vi "xiC - IMAQ - Main.vi"(8 "error in (no error)":errorcluster, 11 "xiCam":refnum<k24>) -> (0 "error out":errorcluster)   [LabVIEW 2013]
doc: "xiControl Main VI. This VI can be used to configure camera parameters and GPI / GPO values.\nThis VI can be called Statically by placing to block diagram or Dynamically with VI server.\n\nCalling this VI with statically connect <b>xiCam</b> parameter for preinited xiCam object, or leave it unwired and the VI automatically initialze a new xiCam object.\n\nDynamic call: Use xiCMNG - Manager VI to handle VI Server call."
uses:
  C:/Projects/Cameras3.x/xiLib/xiLIB_64bit/xiLIB/xiCamLib/API/x64/xiApi.NETX64.dll
  xiLIB_64bit/xiLIB/xiCamLib/API/x64/xiApi.NETX64.dll
  xiCamLib/xiLIB/Typedefs/xiLIB - Control.ctl
  xiCamLib/xiCam/PRM/DOWNSAMPLING_TYPE/DOWNSAMPLING_TYPE.ctl
  xiCamLib/xiCam/PRM/IMG_FORMAT/IMG_DATA_FORMAT.ctl
  xiCamLib/xiCam/PRM/BUFF_POLICY/BUFF_POLICY.ctl
  xiCamLib/xiCam/PRM/TRG_SOURCE/TRG_SOURCE.ctl
  xiCamLib/xiCam/PRM/GPI_MODE/GPI_MODE.ctl
  xiCamLib/xiCam/PRM/GPO_MODE/GPO_MODE.ctl
  xiCamLib/xiCam/PRM/LED_MODE/LED_MODE.ctl
  xiC - IMAQ - States.ctl
  xiC - IMAQ - TreeDisplayType.ctl
  xiCamLib/xiCam/PRM/PRM/PRM_v2.ctl
  xiC - IMAQ - Globals.vi
panel:
  out "Parameter Name":string
  in  "Error":bool=TRUE
  in  "xiControl":T1
  in  "Tree":string(tree)
  out "INFO":string
  in  "RefreshTree":bool
  in  "Stop":bool
  in  "Start":bool
  in  "LOAD":bool
  in  "SAVE":bool
  in  "MANUAL_WB":bool
  in  "SW_TRIG":bool
  in  "GPIO":bool
  out "Image":T9(plugin-control)
  # "xiControl"
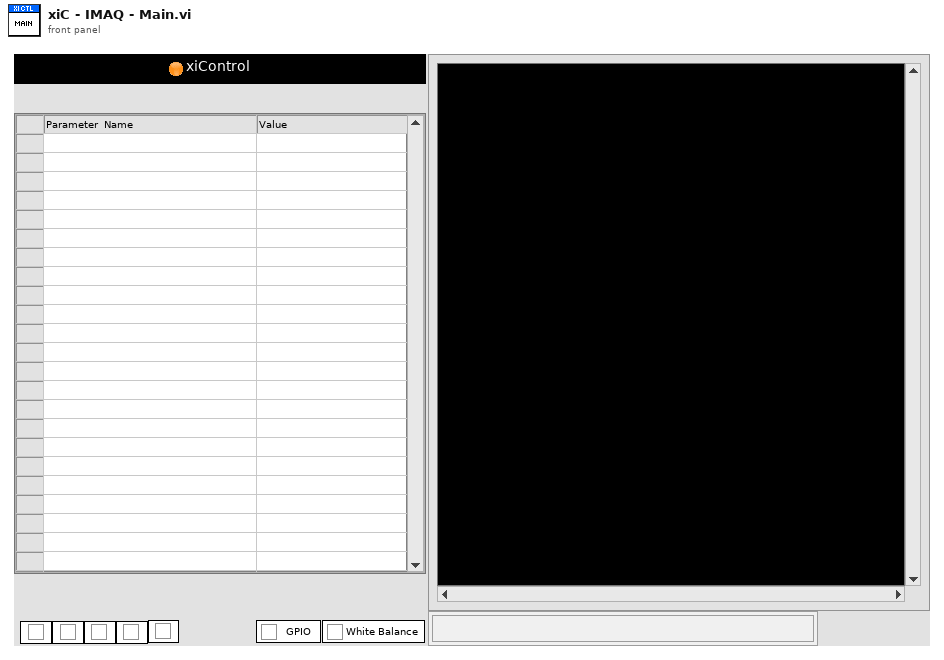
[diagram p1: front panel]
types:
  T1 = typedef "xiLIB - Control.ctl" = cluster{"Int32":i32, "Float":sgl, "String":string, "DOWNSAMPLING_TYPE":T2, "IMG_FORMAT":T3, "BUFF_POLICY":T4, "TRG_SOURCE":T5, "GPI":T6, "GPO":T7, "LED":T8}
  T2 = typedef "DOWNSAMPLING_TYPE.ctl" = enum16{"BINNING", "SKIPPING"}
  T3 = typedef "IMG_DATA_FORMAT.ctl" = enum16{"MONO8", "MONO16", "RGB24", "RGB32", "RGBPLANAR", "RAW8", "RAW16"}
  T4 = typedef "BUFF_POLICY.ctl" = enum16{"UNSAFE", "SAFE"}
  T5 = typedef "TRG_SOURCE.ctl" = enum16{"OFF", "EDGE_RISING", "EDGE_FALLING", "SOFTWARE"}
  T6 = typedef "GPI_MODE.ctl" = enum16{"OFF", "TRIGGER", "EXT_EVENT"}
  T7 = typedef "GPO_MODE.ctl" = enum16{"OFF", "ON", "FRAME_ACTIVE", "FRAME_ACTIVE_NEG", "EXPOSURE_ACTIVE", "EXPOSURE_ACTIVE_NEG"}
  T8 = typedef "LED_MODE.ctl" = enum16{"HEARTBEAT", "TRIGGER_ACTIVE", "EXT_EVENT_ACTIVE", "ACQUSITION", "EXPOSURE_ACTIVE", "FRAME_ACTIVE", "LINK", "OFF", "ON"}
  T9 = typedef "IMAQ Image.ctl" = refnum<image>
  T10 = typedef "xiC - IMAQ - TreeDisplayType.ctl" = enum16{"DEFAULT", "HIDE_MAX_MIN"}
  T11 = typedef "xiC - IMAQ - States.ctl" = enum16{"Idle", "Init", "Exit", "//PRM_UPDATE"}
  T12 = typedef "xiC - IMAQ - Attributes.ctl" = cluster{"Controls":cluster{"VI Ref.":refnum<vi>, "Tree":refnum<vi>, "Info":refnum<vi>, "PRMName":refnum<vi>, "xiControl":refnum<vi>, "Error":refnum<vi>, "SW_TRG":refnum<vi>, "ImageDisplay":refnum<vi>}, "Variables":cluster{"ProcessQ.":refnum<queue>, "Data":bool, "xiCam":refnum<k24>, "Tree_Display_Type":T10}}
  T13 = typedef "PRM_v2.ctl" = enum16{"ACQ_BUFFER_SIZE", "ACQ_FRAME_BURST_COUNT", "ACQ_TIMING_MODE", "ACQ_TRANSPORT_BUFFER_SIZE", "AE_MAX_LIMIT", "AEAG", "AEAG_LEVEL", "API_VERSION", "AG_MAX_LIMIT", "APPLY_CMS", "AUTO_BANDWIDTH_CALCULATION", "AUTO_WB", "AVAILABLE_BANDWIDTH", "AVAILABLE_BANDWIDTH_MAX", "AVAILABLE_BANDWIDTH_MIN", "BPC", "BUFFER_POLICY", "BUFFERS_QUEUE_SIZE", "CC_MATRIX_00", "CC_MATRIX_01", "CC_MATRIX_02", "CC_MATRIX_03", "CC_MATRIX_10", "CC_MATRIX_11", "CC_MATRIX_12", "CC_MATRIX_13", "CC_MATRIX_20", "CC_MATRIX_21", "CC_MATRIX_22", "CC_MATRIX_23", "CC_MATRIX_30", "CC_MATRIX_31", "CC_MATRIX_32", "CC_MATRIX_33", "CHIP_TEMP", "CMS", "COLOR_FILTER_ARRAY", "COOLING", "DEBOUNCE_EN", "DEBOUNCE_POL", "DEBOUNCE_T0", "DEBOUNCE_T1", "DEBUG_LEVEL", "DEFAULT_CC_MATRIX", "DEVICE_INSTANCE_PATH", "DEVICE_MODEL_ID", "DEVICE_NAME", "DEVICE_SN", "DEVICE_TYPE", "DEVICE_USER_ID", "DOWNSAMPLING", "DOWNSAMPLING_MAX", "DOWNSAMPLING_MIN", "DOWNSAMPLING_TYPE", "DRV_VERSION", "EXP_PRIORITY", "EXPOSURE", "EXPOSURE_DIRECT_UPDATE", "EXPOSURE_MAX", "EXPOSURE_MIN", "FFS_FILE_NAME", "FPGA1_VERSION", "FRAMERATE", "FRAMERATE_MAX", "FRAMERATE_MIN", "FREE_FFS_SIZE", "GAIN", "GAIN_DIRECT_UPDATE", "GAIN_MAX", "GAIN_MIN", "GAMMAC", "GAMMAY", "GPI_LEVEL", "GPI_MODE", "GPI_SELECTOR", "GPI_SELECTOR_MAX", "GPI_SELECTOR_MIN", "GPO_MODE", "GPO_SELECTOR", "GPO_SELECTOR_MAX", "GPO_SELECTOR_MIN", "HDR", "HDR_T1", "HDR_T2", "HEIGHT", "HEIGHT_MAX", "HEIGHT_MIN", "HOUSE_TEMP", "IMAGE_DATA_FORMAT", "IMAGE_IS_COLOR", "INPUT_CMS_PROFILE", "IS_COOLED", "IS_DEVICE_EXIST", "KNEEPOINT1", "KNEEPOINT2", "LED_MODE", "LED_SELECTOR", "LED_SELECTOR_MAX", "LED_SELECTOR_MIN", "LIMIT_BANDWIDTH", "LIMIT_BANDWIDTH_MAX", "LIMIT_BANDWIDTH_MIN", "LUT_EN", "LUT_INDEX", "LUT_INDEX_MAX", "LUT_INDEX_MIN", "LUT_VALUE", "LUT_VALUE_MAX", "LUT_VALUE_MIN", "MANUAL_WB", "MCU1_VERSION", "MCU2_VERSION", "OFFSET_X", "OFFSET_X_MAX", "OFFSET_X_MIN", "OFFSET_Y", "OFFSET_Y_MAX", "OFFSET_Y_MIN", "OUTPUT_CMS_PROFILE", "OUTPUT_DATA_BIT_DEPTH", "OUTPUT_DATA_PACKING", "READ_FILE_FFS", "RECENT_FRAME", "SENSOR_DATA_BIT_DEPTH", "SENSOR_MODE", "SENSOR_TAPS", "SHARPNESS", "SHUTTER_TYPE", "TARGET_TEMP", "TRG_DELAY", "TRG_SELECTOR", "TRG_SOFTWARE", "TRG_SOURCE", "USED_FFS_SIZE", "WB_KB", "WB_KG", "WB_KR", "WIDTH", "WIDTH_MAX", "WIDTH_MIN", "WRITE_FILE_FFS", "ACQ_BUFFER_SIZE_UNIT", "ACQ_TRANSPORT_BUFFER_COMMIT", "AEAG_ROI_HEIGHT", "AEAG_ROI_OFFSET_X", "AEAG_ROU_OFFSET_Y", "AEAG_ROI_WIDTH", "API_CONTEXT_LIST", "BINNING_HORIZONTAL", "BINNING_PATTERN", "BINNING_SELECTOR", "BINNING_VERTICAL", "COLUMN_FPN_CORRECTION", "COUNTER_SELECTOR", "COUNTER_VALUE", "DECIMATION_HORIZONTAL", "DECIMATION_PATTERN", "DECIMATION_SELECTOR", "DECIMATION_VERTICAL", "DEVICE_ID", "DEVICE_LOCATION_PATH", "DEVICE_MANIFEST", "DEVICE_RESET", "DEVICE_SENS_SN", "EXPOSURE_BURST_COUNT", "FFS_ACCESS_KEY", "GAIN_SELECTOR", "HW_REVISION", "IMAGE_BLACK_LEVEL", "IMAGE_DATA_BIT_DEPTH", "IMAGE_DATA_FORMAT_RGB32_ALPHA", "IMAGE_PAYLOAD_SIZE", "LENS_APERTURE_VALUE", "LENS_FEATURE", "LENS_FEATURE_SELECTOR", "LENS_FOCAL_LENGTH", "LENS_FOCUS_DISTANCE", "LENS_FOCUS_MOVE", "LENS_FOCUS_MOVEMENT_VALUE", "LENS_MODE", "OUTPUT_DATA_PACKING_TYPE", "SENSOR_CLOCK_FREQ_HZ", "SENSOR_CLOCK_FREQ_INDEX", "SENSOR_FEATURE_SELECTOR", "SENSOR_FEATURE_VALUE", "SENSOR_OUTPUT_CHANNEL_COUNT", "TRANSPORT_PIXEL_FORMAT", "TS_RST_MODE", "TS_RST_SOURCE"}
  T14 = typedef "LVPoint32TypeDef.ctl" = cluster{"Horizontal":i32, "Vertical":i32}
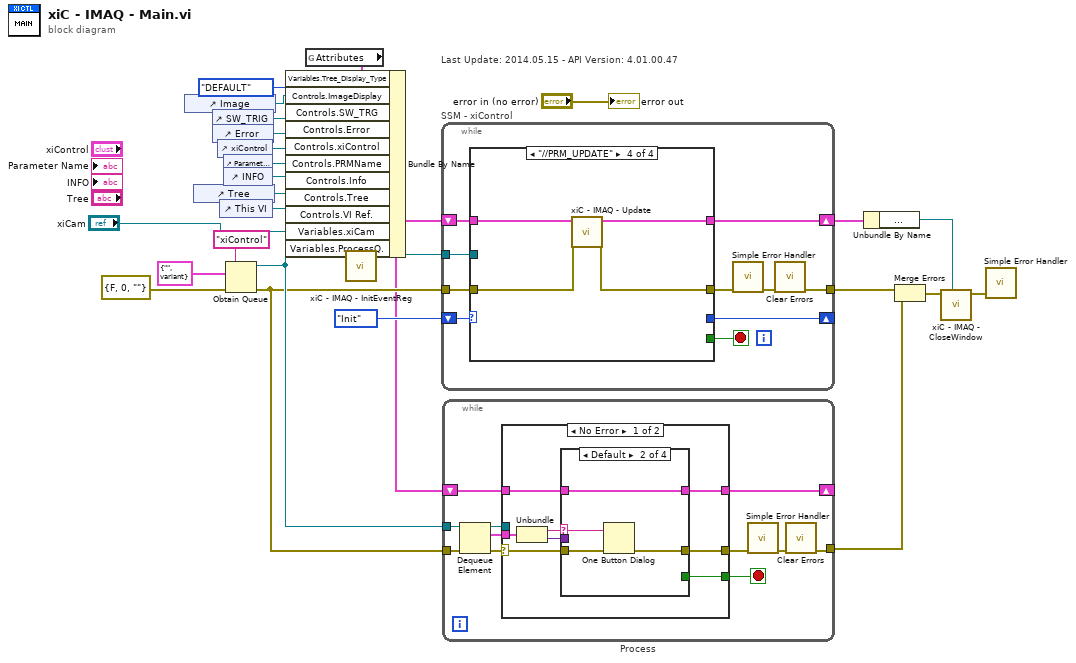
[diagram p0: block diagram]
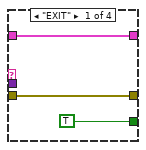
[diagram p2: hidden frame]
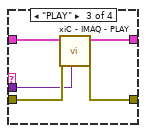
[diagram p3: hidden frame]
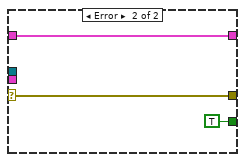
[diagram p5: hidden frame]
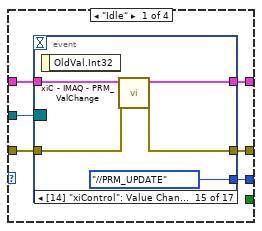
[diagram p6: hidden frame]
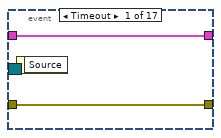
[diagram p7: hidden frame]
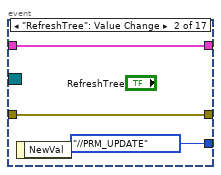
[diagram p8: hidden frame]
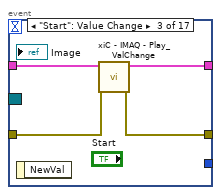
[diagram p9: hidden frame]
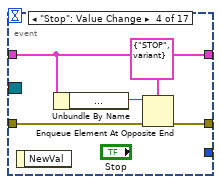
[diagram p10: hidden frame]
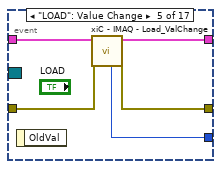
[diagram p11: hidden frame]
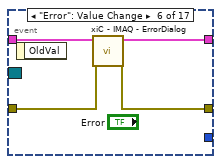
[diagram p12: hidden frame]
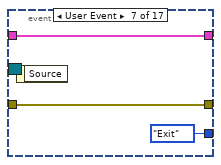
[diagram p13: hidden frame]
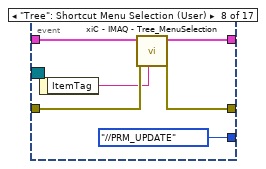
[diagram p14: hidden frame]
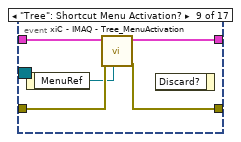
[diagram p15: hidden frame]
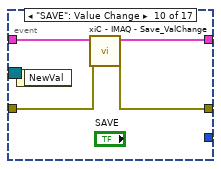
[diagram p16: hidden frame]
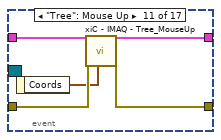
[diagram p17: hidden frame]
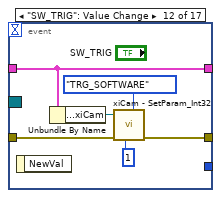
[diagram p18: hidden frame]
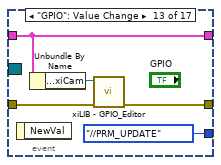
[diagram p19: hidden frame]
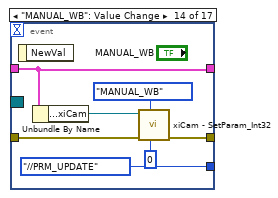
[diagram p20: hidden frame]
diagram:
  # "Last Update: 2014.05.15 - API Version: 4.01.00.47"
  n1 = control-ref of="Image"() -> (w3:refnum<vi>)
  n2 = control-ref of="Tree"() -> (w21:refnum<vi>)
  n3 = control-ref of="SW_TRIG"() -> (w14:refnum<vi>)
  n4 = control-ref of="Error"() -> (w15:refnum<vi>)
  n5 = control-ref of="xiControl"() -> (w1:refnum<vi>)
  n6 = control-ref of="This VI"() -> (w25:refnum<vi>)
  n7 = control-ref of="Parameter Name"() -> (w17:refnum<vi>)
  n8 = control-ref of="INFO"() -> (w18:refnum<vi>)
  n9 = Obtain Queue(name (unnamed)="xiControl", element data type=cluster{"State":string, "Data":variant} {"State"="", "Data"=variant} ("element"), error in (no error)=errorcluster {"status"=FALSE, "code"=0, "source"=""}) -> (queue out=w7:refnum<queue>, error out=w6:errorcluster)  [unwired: 2 in, 1 out]
  n10 = global read "xiC - IMAQ - Globals.vi" "Attributes"() -> (w16:T12)
  n11 = Bundle By Name(cluster=w16, "Variables.Tree_Display_Type"=xiC_-_IMAQ_-_TreeDisplayType."DEFAULT" ("Variables.SAVE_Type"), "Controls.ImageDisplay"=w3, "Controls.SW_TRG"=w14, "Controls.Error"=w15, "Controls.xiControl"=w1, "Controls.PRMName"=w17, "Controls.Info"=w18, "Controls.Tree"=w21, "Controls.VI Ref."=w25, "Variables.xiCam"="xiCam", "Variables.ProcessQ."=w7) -> (w5:T12)
  n12 = call "xiC - IMAQ - InitEventReg.vi"() -> ("EventRegRef"=w13:refnum<event-registration>)  [unwired: 11 in]
  n13 = while "SSM - xiControl" {
    shift-right: [w30] -> _
    shift-left: xiC_-_IMAQ_-_States."Init" ("States") -> [w36]
    shift-right: [w34] -> w23
    shift-left: w5 -> [w35]
    tunnel: w6 -> [w33]
    tunnel: [w31] -> w12
    tunnel: w13 -> [w28]
    stop <- w29 stop-if-true
    n14 = case shown="\"//PRM_UPDATE\"" w36 {
      tunnel: w35 -> [w42 w126 w130 w136]
      tunnel: [w41 w125 w128 w135] -> w34
      tunnel: w33 -> [w40 w124 w129 w134]
      tunnel: [w39 w120 w127 w133] -> w27
      tunnel: [w38 w121 xiC_-_IMAQ_-_States."Exit" ("States") _] -> w30
      tunnel: [_ _ TRUE _] -> w29
      tunnel: w28 -> [w37 _ _ _]
      frame "Idle" {
        n15 = event shown="[14] \"xiControl\": Value Change" {
          selector: w37 -> [_ _ _ _ _ _ _ _ _ _ _ _ _ _ _ _ _]
          dyn-events: _ -> [_ _ _ _ _ _ _ _ _ _ _ _ _ _ _ _ _]
          timeout: _ -> [_ _ _ _ _ _ _ _ _ _ _ _ _ _ _ _ _]
          tunnel: w42 -> [w44 w47 w51 w52 w61 w65 w68 w74 w79 w83 w88 w94 w96 w101 w111 w115 w119]
          tunnel: [w44 w47 w50 w52 w60 w64 w68 w73 w78 w82 w87 w94 w96 w101 w110 w114 w119] -> w41
          tunnel: w40 -> [w43 w46 w49 w54 w59 w63 w67 w72 w77 w81 w86 w92 w99 w103 w109 w113 w117]
          tunnel: [w43 w46 w48 w53 w58 w62 w67 w71 w76 w80 w85 w91 w98 w102 w108 w112 w117] -> w39
          tunnel: [_ xiC_-_IMAQ_-_States."//PRM_UPDATE" ("States") _ _ w57 _ xiC_-_IMAQ_-_States."Exit" ("States") xiC_-_IMAQ_-_States."//PRM_UPDATE" ("States") _ _ _ _ xiC_-_IMAQ_-_States."//PRM_UPDATE" ("States") xiC_-_IMAQ_-_States."//PRM_UPDATE" ("States") xiC_-_IMAQ_-_States."//PRM_UPDATE" ("States") _ xiC_-_IMAQ_-_States."Exit" ("States")] -> w38
          event Timeout {
            n16 = event-data() -> ()  [unwired: 1 in, 1 out]
          }
          event "RefreshTree": Value Change {
            n17 = event-data() -> ()  [unwired: 1 in, 1 out]
          }
          event "Start": Value Change {
            n18 = event-data() -> ()  [unwired: 1 in, 1 out]
            n19 = call "xiC - IMAQ - Play_ValChange.vi"("error in (no error)"=w49, "Attributes In"=w51) -> ("error out"=w48:errorcluster, "Attributes Out"=w50:T12)  [unwired: 8 in]
          }
          event "Stop": Value Change {
            n20 = event-data() -> ()  [unwired: 1 in, 1 out]
            n21 = Unbundle By Name(w52) -> ("Variables.ProcessQ."=w55:refnum<queue>)
            n22 = Enqueue Element At Opposite End(queue=w55, element=cluster{"State":string, "Data":variant} {"State"="STOP", "Data"=variant}, error in (no error)=w54) -> (error out=w53:errorcluster)  [unwired: 1 in, 2 out]
          }
          event "LOAD": Value Change {
            n23 = event-data() -> ()  [unwired: 1 in, 1 out]
            n24 = call "xiC - IMAQ - Load_ValChange.vi"("error in (no error)"=w59, "Attributes In"=w61) -> ("error out"=w58:errorcluster, "Attributes Out"=w60:T12, "State"=w57:T11)  [unwired: 7 in]
          }
          event "Error": Value Change {
            n25 = event-data() -> ()  [unwired: 1 in, 1 out]
            n26 = call "xiC - IMAQ - ErrorDialog.vi"("error in (no error)"=w63, "Attributes In"=w65) -> ("error out"=w62:errorcluster, "Attributes Out"=w64:T12)  [unwired: 8 in]
          }
          event User Event {
            n27 = event-data() -> ()  [unwired: 1 in, 1 out]
          }
          event "Tree": Shortcut Menu Selection (User) {
            n28 = event-data() -> ("ItemTag"=w70:string)  [unwired: 1 in]
            n29 = call "xiC - IMAQ - Tree_MenuSelection.vi"("SelectedMenuTag"=w70, "error in (no error)"=w72, "Attributes In"=w74) -> ("error out"=w71:errorcluster, "Attributes Out"=w73:T12)  [unwired: 7 in]
          }
          event "Tree": Shortcut Menu Activation? {
            n30 = event-data() -> ("MenuRef"=w75:refnum<k9>)  [unwired: 1 in]
            n31 = call "xiC - IMAQ - Tree_MenuActivation.vi"("Menu Refnum"=w75, "error in (no error)"=w77, "Attributes In"=w79) -> ("error out"=w76:errorcluster, "Attributes Out"=w78:T12)  [unwired: 7 in]
            n32 = event-data() -> ()  [unwired: 2 in, 1 out]
          }
          event "SAVE": Value Change {
            n33 = event-data() -> ()  [unwired: 1 in, 1 out]
            n34 = call "xiC - IMAQ - Save_ValChange.vi"("error in (no error)"=w81, "Attributes In"=w83) -> ("error out"=w80:errorcluster, "Attributes Out"=w82:T12)  [unwired: 8 in]
          }
          event "Tree": Mouse Up {
            n35 = event-data() -> ("Coords"=w84:T14)  [unwired: 1 in]
            n36 = call "xiC - IMAQ - Tree_MouseUp.vi"("Coords"=w84, "error in (no error)"=w86, "Attributes In"=w88) -> ("error out"=w85:errorcluster, "Attributes Out"=w87:T12)  [unwired: 7 in]
          }
          event "SW_TRIG": Value Change {
            n37 = event-data() -> ()  [unwired: 1 in, 1 out]
            n38 = Unbundle By Name(w94) -> ("Variables.xiCam"=w93:refnum<k24>)
            n39 = call "xiCam - SetParam_Int32.vi"("Int32_Value"=1, "PRM"=PRM_v2."TRG_SOFTWARE", "error in (no error)"=w92, "xiCam In"=w93) -> ("error out"=w91:errorcluster)  [unwired: 6 in, 1 out]
          }
          event "GPIO": Value Change {
            n40 = event-data() -> ()  [unwired: 1 in, 1 out]
            n41 = Unbundle By Name(w96) -> ("Variables.xiCam"=w95:refnum<k24>)
            n42 = call "xiLIB - GPIO_Editor.vi"("error in (no error)"=w99, "xiCam In"=w95) -> ("error out"=w98:errorcluster)  [unwired: 9 in]
          }
          event "MANUAL_WB": Value Change {
            n43 = event-data() -> ()  [unwired: 1 in, 1 out]
            n44 = Unbundle By Name(w101) -> ("Variables.xiCam"=w104:refnum<k24>)
            n45 = call "xiCam - SetParam_Int32.vi"("Int32_Value"=0, "PRM"=PRM_v2."MANUAL_WB", "error in (no error)"=w103, "xiCam In"=w104) -> ("error out"=w102:errorcluster)  [unwired: 6 in, 1 out]
          }
          event Value Change {
            n46 = event-data() -> ()  [unwired: 1 in, 1 out]
            n47 = call "xiC - IMAQ - PRM_ValChange.vi"("error in (no error)"=w109, "Attributes In"=w111) -> ("error out"=w108:errorcluster, "Attributes Out"=w110:T12)  [unwired: 8 in]
          }
          event "Tree": Value Change {
            n48 = event-data() -> ()  [unwired: 1 in, 1 out]
            n49 = call "xiC - IMAQ - Tree_ValChange.vi"("error in (no error)"=w113, "Attributes In"=w115) -> ("error out"=w112:errorcluster, "Attributes Out"=w114:T12)  [unwired: 8 in]
          }
          event Panel Close? {
            n50 = event-data() -> ()  [unwired: 1 in, 1 out]
            n51 = event-data("Discard?"=TRUE) -> ()  [unwired: 1 in, 1 out]
          }
        }
      }
      frame "Init" {
        n52 = call "xiC - IMAQ - Init.vi"("error in (no error)"=w124, "Attributes In"=w126) -> ("error out"=w120:errorcluster, "Attributes Out"=w125:T12)  [unwired: 8 in]
        n53 = Select(t=xiC_-_IMAQ_-_States."Exit" ("States"), s=w120, f=xiC_-_IMAQ_-_States."//PRM_UPDATE" ("States")) -> (s? t:f=w121:T11)
      }
      frame "Exit" {
        n54 = call "xiC - IMAQ - Exit.vi"("error in (no error)"=w129, "Attributes In"=w130) -> ("error out"=w127:errorcluster, "Attributes Out"=w128:T12)  [unwired: 8 in]
      }
      frame "//PRM_UPDATE" {
        n55 = call "xiC - IMAQ - Update.vi"("error in (no error)"=w134, "Attributes In"=w136) -> ("error out"=w133:errorcluster, "Attributes Out"=w135:T12)  [unwired: 8 in]
      }
    }
    n56 = call <vilib>:"Simple Error Handler.vi"("error in (no error)"=w27) -> ("error out"=w32:errorcluster)  [unwired: 4 in, 4 out]
    n57 = call <vilib>:"Clear Errors.vi"("error in (no error)"=w32) -> ("error out"=w31:errorcluster)  [unwired: 6 in]
  }
  n58 = while "Process" {
    tunnel: [w143] -> w4
    tunnel: w6 -> [w141]
    tunnel: w7 -> [w140]
    shift-right: [w138] -> _
    shift-left: w5 -> [w139]
    stop <- w142 stop-if-true
    n59 = Dequeue Element(queue=w140, error in (no error)=w141) -> (queue out=w146:refnum<queue>, element=w145:cluster{"State":string, "Data":variant}, error out=w147:errorcluster)  [unwired: 1 in, 1 out]
    n60 = case shown="No Error" w147 {
      selector: w147 -> [w152 w171]
      tunnel: w146 -> [_ _]
      tunnel: w145 -> [w155 _]
      tunnel: [w151 w171] -> w137
      tunnel: [w150 TRUE] -> w142
      tunnel: w139 -> [w149 w170]
      tunnel: [w148 w170] -> w138
      frame No Error {
        n61 = Unbundle(w155) -> ("State"=w154:string, "Data"=w153:variant)
        n62 = case shown="Default" w154 {
          selector: w154 -> [_ w161 _ _]
          tunnel: w153 -> [_ _ w162 _]
          tunnel: w152 -> [w157 w160 w164 w167]
          tunnel: [w157 w160 w163 w167] -> w151
          tunnel: [TRUE _ _ _] -> w150
          tunnel: w149 -> [w156 w159 w166 w168]
          tunnel: [w156 w159 w165 w168] -> w148
          frame "EXIT" {
          }
          frame Default {
            n63 = One Button Dialog(message=w161) -> ()  [unwired: 1 in, 1 out]
          }
          frame "PLAY" {
            n64 = call "xiC - IMAQ - PLAY.vi"("Data"=w162, "error in (no error)"=w164, "Attributes In"=w166) -> ("error out"=w163:errorcluster, "Attributes In"=w165:T12)  [unwired: 7 in]
          }
          frame "STOP" {
          }
        }
      }
      frame Error {
      }
    }
    n65 = call <vilib>:"Simple Error Handler.vi"("error in (no error)"=w137) -> ("error out"=w144:errorcluster)  [unwired: 4 in, 4 out]
    n66 = call <vilib>:"Clear Errors.vi"("error in (no error)"=w144) -> ("error out"=w143:errorcluster)  [unwired: 6 in]
  }
  n67 = Unbundle By Name(w23) -> ("Controls.VI Ref."=w22:refnum<vi>)
  n68 = Merge Errors(w12, w4) -> (w11:errorcluster)
  n69 = call "xiC - IMAQ - CloseWindow.vi"("VI Refnum"=w22, "error in (no error)"=w11) -> ("error out"=w24:errorcluster)  [unwired: 9 in]
  n70 = call <vilib>:"Simple Error Handler.vi"("error in (no error)"=w24) -> ()  [unwired: 4 in, 5 out]
  "error out" <- "error in (no error)"
